vi "Close.vi"(8 "error in (no error)":errorcluster, 11 "FPGA_Sim in":refnum<class "FPGA_Mock.lvclass">) -> (0 "error out":errorcluster, 3 "FPGA_Sim out":refnum<class "FPGA_Mock.lvclass">)   [LabVIEW 2019, in "FPGA_Mock.lvclass"]
uses:
  FPGA_Mock.lvclass
  FPGA_Mock.lvclass/FPGA_Mock.ctl
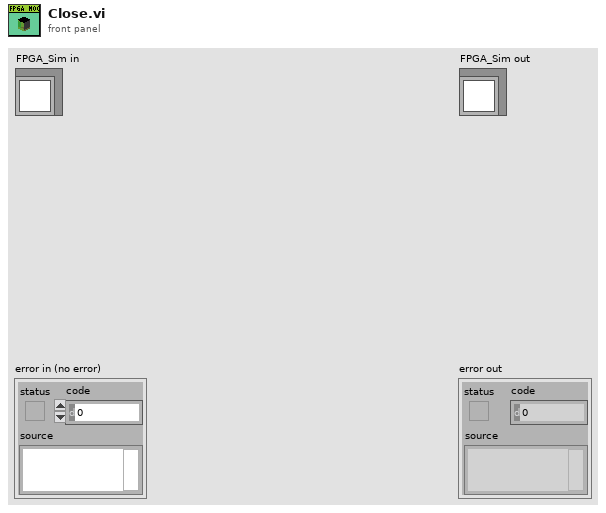
[diagram p1: front panel]
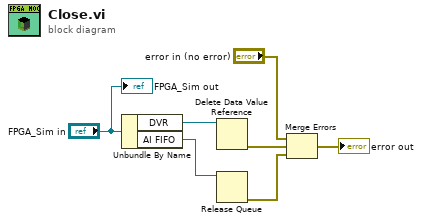
[diagram p0: block diagram]
diagram:
  n1 = Unbundle By Name("FPGA_Sim in") -> ("DVR"=w6:refnum<data-value>, "AI FIFO"=w5:refnum<queue>)
  n2 = Delete Data Value Reference(data value reference=w6) -> (error out=w4:errorcluster)  [unwired: 1 in, 1 out]
  n3 = Release Queue(queue=w5) -> (error out=w3:errorcluster)  [unwired: 2 in, 2 out]
  n4 = Merge Errors("error in (no error)", w4, w3) -> (→"error out":errorcluster)
  "FPGA_Sim out" <- "FPGA_Sim in"
